vi "Find Longest Line.vi"(10 "Array":cluster{i32[]}[](array[cluster])) -> (2 "Edge":cluster{"Column":i32, "Row":i32}[](array[cluster]))   [LabVIEW 2013]
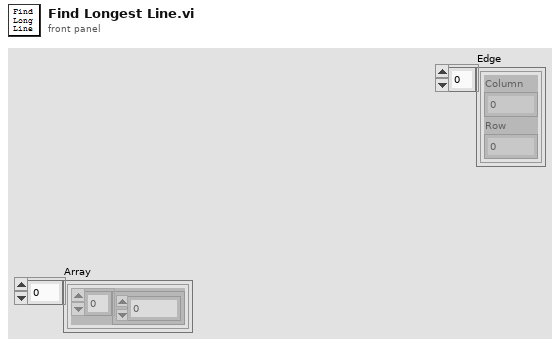
[diagram p1: front panel]
types:
  T1 = cluster{"Length":i32, "Head":cluster{"Column":i32, "Row":i32}, "Current Row":i32, "Points":cluster{"Column":i32, "Row":i32}[]}[]
  T2 = cluster{"Length":i32, "Head":cluster{"Column":i32, "Row":i32}, "Current Row":i32, "Points":cluster{"Column":i32, "Row":i32}[]}
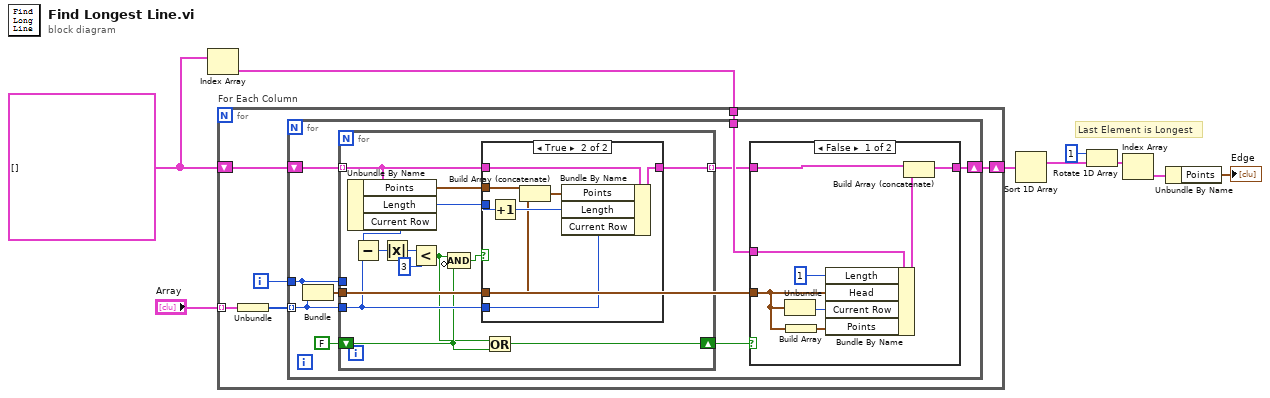
[diagram p0: block diagram]
diagram:
  w8 = T1 []
  # "Last Element is Longest"
  n1 = Index Array(array=w8) -> (element=w7:T2)  [unwired: 1 in]
  n2 = for "For Each Column" {
    tunnel: "Array" -> [w15] mode=indexing
    shift-right: [w12] -> w6
    shift-left: w8 -> [w10]
    tunnel: w7 -> [w13]
    i -> [w14]
    n3 = Unbundle(w15) -> (w11:i32[])
    n4 = for {
      tunnel: w11 -> [w21] mode=indexing
      shift-right: [w24] -> w12
      shift-left: w10 -> [w17]
      tunnel: w14 -> [w22]
      tunnel: w13 -> [w23]
      n5 = Bundle(w22, w21) -> (w20:cluster{i32, i32})  [unwired: 1 in]
      n6 = for {
        tunnel: w17 -> [w43] mode=indexing
        tunnel: [w41] -> w18 mode=indexing
        tunnel: w21 -> [w40]
        tunnel: w22 -> [_]
        tunnel: w20 -> [w38]
        shift-right: [w37] -> w19
        shift-left: FALSE -> [w36]
        n7 = Unbundle By Name(w43) -> ("Points"=w39:cluster{"Column":i32, "Row":i32}[], "Length"=w42:i32, "Current Row"=w47:i32)
        n8 = Subtract(x=w47, y=w40) -> (x-y=w46:i32)
        n9 = Absolute Value(x=w46) -> (abs(x)=w45:i32)
        n10 = Less?(x=w45, y=3) -> (x < y?=w35:bool)
        n11 = Compound Arithmetic op=AND(w35, invert w36) -> (w34:bool)
        n12 = case shown="True" w34 {
          tunnel: w43 -> [w48 w55]
          tunnel: w42 -> [_ w56]
          tunnel: [w48 w54] -> w41
          tunnel: w40 -> [_ w52]
          tunnel: w39 -> [_ w51]
          tunnel: w38 -> [_ w49]
          frame False {
          }
          frame True {
            n13 = Increment(x=w56) -> (x+1=w53:i32)
            n14 = Build Array (concatenate)(w51, w49) -> (w50:cluster{"Column":i32, "Row":i32}[])
            n15 = Bundle By Name(cluster=w55, "Points"=w50, "Length"=w53, "Current Row"=w52) -> (w54:T2)
          }
        }
        n16 = Or(x=w35, y=w36) -> (x .or. y?=w37:bool)
      }
      n17 = case shown="False" w19 {
        tunnel: w18 -> [w26 w33]
        tunnel: [w25 w33] -> w24
        tunnel: w23 -> [w32 _]
        tunnel: w20 -> [w29 _]
        frame False {
          n18 = Unbundle(w29) -> (w28:i32)  [unwired: 1 out]
          n19 = Build Array(w29) -> (w30:cluster{i32, i32}[])
          n20 = Bundle By Name(cluster=w32, "Length"=1, "Head"=w29, "Current Row"=w28, "Points"=w30) -> (w27:T2)
          n21 = Build Array (concatenate)(w26, w27) -> (w25:T1)
        }
        frame True {
        }
      }
    }
  }
  n22 = Sort 1D Array(array=w6) -> (sorted array=w5:T1)
  n23 = Rotate 1D Array(1:w5, 2:1 ("n")) -> (0:w4:T1)
  n24 = Index Array(array=w4) -> (element=w2:T2)  [unwired: 1 in]
  n25 = Unbundle By Name(w2) -> ("Points"=→"Edge":cluster{"Column":i32, "Row":i32}[])
